vi "rd_initialFormat.vi"(4 "data type":T1, 6 "column index":i32, 8 "error in (no error)":errorcluster, 9 "column format":string, 10 "TimeColumnMode":T2, 11 "TimestampFormat":string) -> (0 "error out":errorcluster, 3 "column format out":string)   [LabVIEW 2020, in "NI_ExcelFile.lvlib"]
uses:
  <vilib>/express/express shared/NI_ExcelFile/NI_ExcelFile.lvlib
  <vilib>/express/express shared/NI_ExcelFile/Ctrls/TimeColumnMode.ctl
  <vilib>/express/express shared/NI_ExcelFile/Ctrls/DataType.ctl
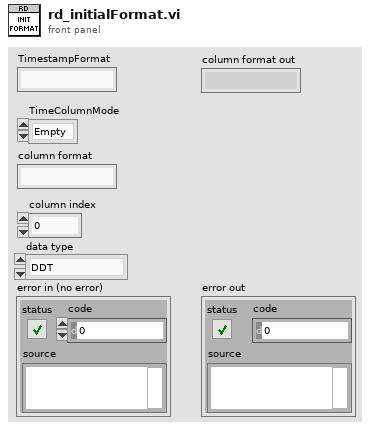
[diagram p1: front panel]
types:
  T1 = typedef "NI_ExcelFile.lvlib/DataType.ctl" = enum16{"DDT", "WFM", "Array of STR", "Array of DBL", "Array of I8", "Array of I16", "Array of I32", "Array of I64", "Array of SGL", "Array of U8", "Array of U16", "Array of U32", "Array of U64", "Array of Time"}
  T2 = typedef "NI_ExcelFile.lvlib/TimeColumnMode.ctl" = enum16{"Empty", "OnePerCh", "One"}
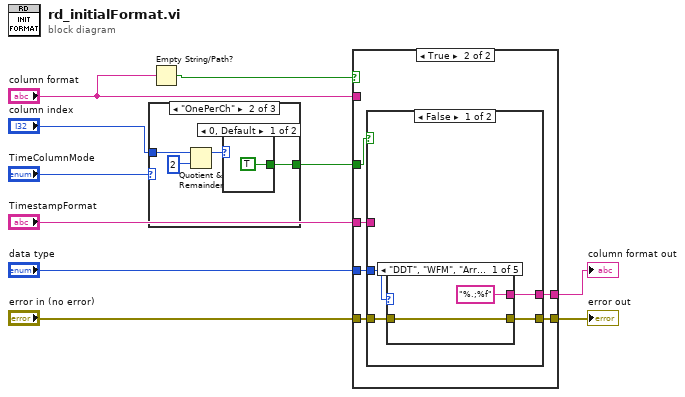
[diagram p0: block diagram]
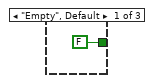
[diagram p2: hidden frame]
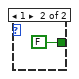
[diagram p3: hidden frame]
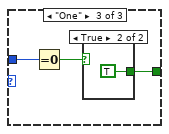
[diagram p4: hidden frame]
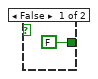
[diagram p5: hidden frame]
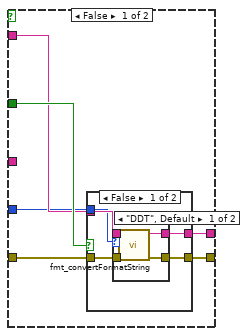
[diagram p6: hidden frame]
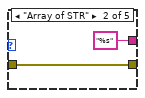
[diagram p9: hidden frame]
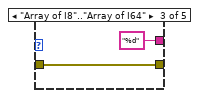
[diagram p10: hidden frame]
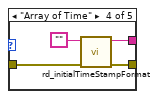
[diagram p11: hidden frame]
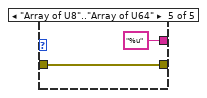
[diagram p12: hidden frame]
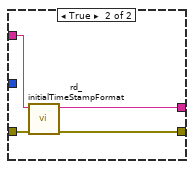
[diagram p13: hidden frame]
diagram:
  n1 = case shown="\"OnePerCh\"" "TimeColumnMode" {
    tunnel: "column index" -> [_ w13 w19]
    tunnel: [FALSE w12 w18] -> w3
    frame "Empty", Default {
    }
    frame "OnePerCh" {
      n2 = Quotient & Remainder(x=w13, y=2) -> (x-y*floor(x/y)=w14:i32)  [unwired: 1 out]
      n3 = case shown="0, Default" w14 {
        tunnel: [TRUE FALSE] -> w12
        frame 0, Default {
        }
        frame 1 {
        }
      }
    }
    frame "One" {
      n4 = Equal To 0?(x=w19) -> (x = 0?=w20:bool)
      n5 = case shown="True" w20 {
        tunnel: [FALSE TRUE] -> w18
        frame False {
        }
        frame True {
        }
      }
    }
  }
  n6 = Empty String/Path?(string/path="column format") -> (empty?=w7:bool)
  n7 = case shown="True" w7 {
    tunnel: "error in (no error)" -> [w26 w47]
    tunnel: "column format" -> [w27 _]
    tunnel: [w24 w45] -> w5
    tunnel: "TimestampFormat" -> [_ w43]
    tunnel: "data type" -> [w23 w46]
    tunnel: w3 -> [w28 w42]
    tunnel: [w25 w44] -> w2
    frame False {
      n8 = case shown="False" w28 {
        tunnel: w27 -> [w33 w40]
        tunnel: w26 -> [w32 w41]
        tunnel: [w31 w41] -> w25
        tunnel: [w30 w40] -> w24
        tunnel: w23 -> [w29 _]
        frame False {
          n9 = case shown="\"DDT\", Default" w29 {
            tunnel: w33 -> [w37 w39]
            tunnel: w32 -> [w36 w38]
            tunnel: [w35 w38] -> w31
            tunnel: [w34 w39] -> w30
            frame "DDT", Default {
              n10 = call <vilib>:"fmt_convertFormatString.vi"("error in (no error)"=w36, "format string"=w37) -> ("error out"=w35:errorcluster, "format string out"=w34:string)  [unwired: 8 in]
            }
            frame "Array of Time" {
            }
          }
        }
        frame True {
        }
      }
    }
    frame True {
      n11 = case shown="False" w42 {
        tunnel: w47 -> [w50 w67]
        tunnel: w46 -> [w51 _]
        tunnel: [w49 w65] -> w45
        tunnel: [w48 w66] -> w44
        tunnel: w43 -> [_ w64]
        frame False {
          n12 = case shown="\"DDT\", \"WFM\", \"Array of DBL\", \"Array of SGL\", Default" w51 {
            tunnel: ["%.;%f" "%s" "%d" w61 "%u"] -> w49
            tunnel: w50 -> [w52 w54 w56 w59 w62]
            tunnel: [w52 w54 w56 w58 w62] -> w48
            frame "DDT", "WFM", "Array of DBL", "Array of SGL", Default {
            }
            frame "Array of STR" {
            }
            frame "Array of I8".."Array of I64" {
            }
            frame "Array of Time" {
              n13 = call <vilib>:"rd_initialTimeStampFormat.vi"("error in (no error)"=w59, "timestamp format"="") -> ("error out"=w58:errorcluster, "timestamp format out"=w61:string)  [unwired: 8 in]
            }
            frame "Array of U8".."Array of U64" {
            }
          }
        }
        frame True {
          n14 = call <vilib>:"rd_initialTimeStampFormat.vi"("error in (no error)"=w67, "timestamp format"=w64) -> ("error out"=w66:errorcluster, "timestamp format out"=w65:string)  [unwired: 8 in]
        }
      }
    }
  }
  "error out" <- w2
  "column format out" <- w5
